vi "write_to_file.vi"(8 "data 3":bool[](array[boolean]), 11 "file (use dialog) in":path) -> ()   [LabVIEW 2013]
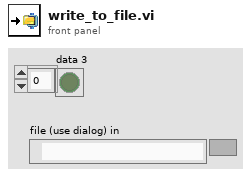
[diagram p1: front panel]
types:
  T1 = enum16{"open", "replace", "create", "open or create", "replace or create", "replace or create with confirmation"}
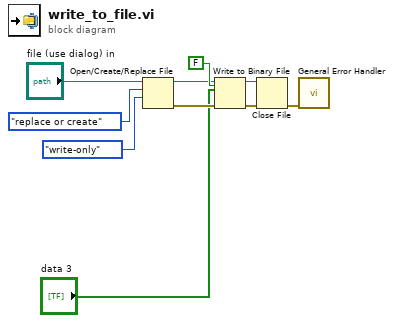
[diagram p0: block diagram]
diagram:
  n1 = Open/Create/Replace File(file path (use dialog)="file (use dialog) in", operation (0:open)=T1."replace or create", access (0:read/write)=enum16{"read/write", "read-only", "write-only"}."write-only") -> (refnum out=w6:refnum<file>, error out=w4:errorcluster)  [unwired: 3 in, 1 out]
  n2 = Write to Binary File(file (use dialog)=w6, data="data 3", error in=w4, 5:FALSE ("prepend array or string size? (T)")) -> (refnum out=w10:refnum<file>, error out=w3:errorcluster)  [unwired: 2 in, 1 out]
  n3 = Close File(refnum=w10, error in=w3) -> (error out=w2:errorcluster)  [unwired: 1 out]
  n4 = call <vilib>:"General Error Handler.vi"("error in (no error)"=w2) -> ()  [unwired: 10 in, 5 out]
